vi "Select Train Rate.vi"() -> ()   [LabVIEW 2009, in "Power Supply.lvclass"]
uses:
  Power Supply.lvclass
  Power Supply.lvclass/Power Supply.ctl
panel:
  out "going up?":bool
  in  "Rate Out":dbl[unit]=0.11666666666666667
  out "Power Supply Out":refnum<class "Power Supply.lvclass">
  in  "Power Supply in":refnum<class "Power Supply.lvclass">
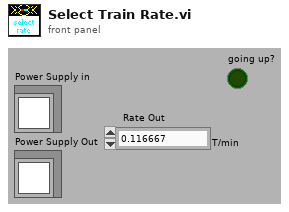
[diagram p1: front panel]
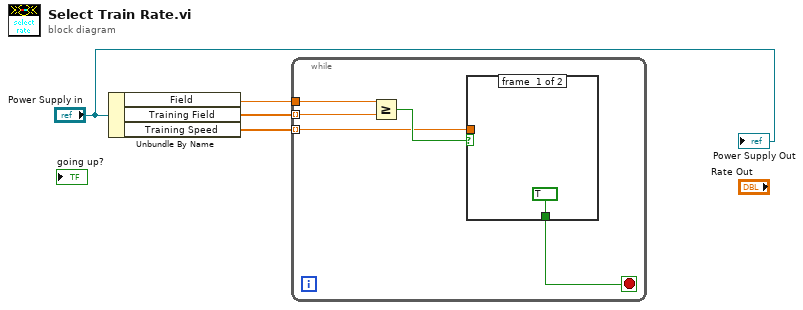
[diagram p0: block diagram]
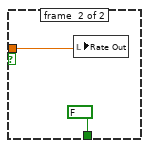
[diagram p2: hidden frame]
diagram:
  n1 = Unbundle By Name("Power Supply in") -> ("Field"=w2:dbl[unit], "Training Field"=w4:dbl[unit][], "Training Speed"=w3:dbl[unit][])
  n2 = while {
    tunnel: w4 -> [w8] mode=indexing
    tunnel: w3 -> [w6] mode=indexing
    tunnel: w2 -> [w9]
    stop <- w5 stop-if-true
    n3 = Greater Or Equal?(x=w9, y=w8) -> (x >= y?=w7:bool)
    n4 = case shown="True" w7 {
      tunnel: w6 -> [_ w12]
      tunnel: [TRUE FALSE] -> w5
      frame #0 {
      }
      frame #1 {
        n5 = local write "Rate Out"(w12) -> ()
      }
    }
  }
  "Power Supply Out" <- "Power Supply in"
